vi "Set Name.vi"(10 "name":string, 11 "Configuration in":refnum<class "Configuration.lvclass">) -> (3 "Configuration out":refnum<class "Configuration.lvclass">)   [LabVIEW 2017, in "Data Sharing Framework Engine.lvlib" / "Configuration.lvclass"]
uses:
  Configuration.lvclass
  Configuration.lvclass/Configuration.ctl
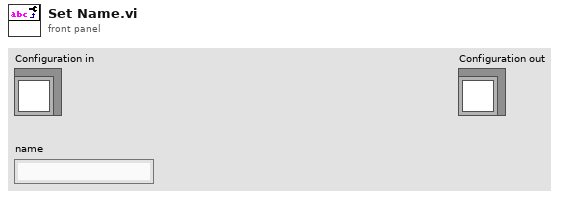
[diagram p1: front panel]
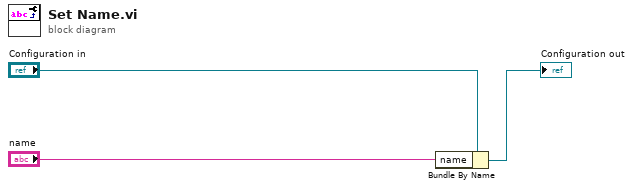
[diagram p0: block diagram]
diagram:
  n1 = Bundle By Name(cluster="Configuration in", "name"="name") -> (→"Configuration out":refnum<class "Configuration.lvclass">)
